vi "xor_block.vi"(2 "Control":T3, 3 "B":T4, 4 "A":T5) -> (0 "Flags":T1, 1 "Result":T2)   [LabVIEW 2013]
panel:
  # "R1"
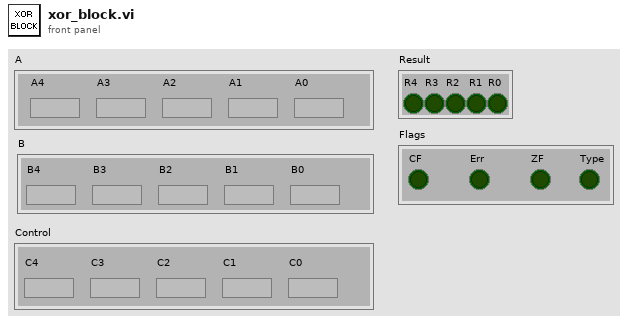
[diagram p1: front panel]
types:
  T1 = cluster{"CF":bool, "Err":bool, "ZF":bool, "Type":bool}
  T2 = cluster{"R4":bool, "R3":bool, "R2":bool, bool, "R0":bool}
  T3 = cluster{"C4":bool, "C3":bool, "C2":bool, "C1":bool, "C0":bool}
  T4 = cluster{"B4":bool, "B3":bool, "B2":bool, "B1":bool, "B0":bool}
  T5 = cluster{"A4":bool, "A3":bool, "A2":bool, "A1":bool, "A0":bool}
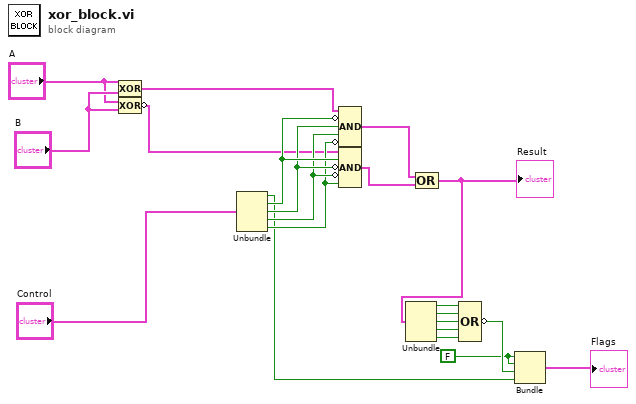
[diagram p0: block diagram]
diagram:
  w6 = FALSE
  n1 = Compound Arithmetic op=XOR("A", "B") -> (w3:cluster{bool, bool, bool, bool, bool})
  n2 = Compound Arithmetic op=XOR("A", "B") -> (invert w2:cluster{bool, bool, bool, bool, bool})
  n3 = Unbundle("Control") -> ("C4"=w1:bool, "C3"=w19:bool, "C2"=w18:bool, "C1"=w17:bool, "C0"=w16:bool)
  n4 = Compound Arithmetic op=AND(w3, invert w19, w18, w17, invert w16) -> (w21:cluster{bool, bool, bool, bool, bool})
  n5 = Compound Arithmetic op=AND(w2, w19, invert w18, invert w17, w16) -> (w20:cluster{bool, bool, bool, bool, bool})
  n6 = Compound Arithmetic op=OR(w21, w20) -> (w13:cluster{bool, bool, bool, bool, bool})
  "Result" <- w13
  n7 = Unbundle(w13) -> (w12:bool, w11:bool, w10:bool, w9:bool, w8:bool)
  n8 = Compound Arithmetic op=OR(w12, w11, w10, w9, w8) -> (invert w7:bool)
  n9 = Bundle(w6, w6, w7, "C4"=w1) -> (→"Flags":cluster{bool, bool, bool, "C4":bool})  [unwired: 1 in]
